vi "Advanced Cut - Remove Snippet Impulse Data.vi"(8 "error in (no error)":errorcluster, 10 "Snippet Domain in (samples)":dbl[](array[numeric]), 11 "Data IN":T1={"Impulse Positions"=[], "No. Imp"=0, "Parameter Time Series"=[], "Parameter Impuls Series"=[], "Experiment Parameters"={"Freq"=0.0, "Vel"=0, "Acc"=0, "Stimulus"=""}, "Autosort File"=refnum, "Data File"={"Data Channels"=[], "Sample Rate"=0, "Channel List"=[]}, "Experiment data path"=path "/Macintosh HD/Users/patrick/Studium/Diploma Thesis/Data Analysis", "Image data path"=path "/Macintosh HD/Users/patrick/Studium/Diploma Thesis/Data Analysis", "LVS data path"=path "/Macintosh HD/Users/patrick/Studium/Diploma Thesis/Data Analysis", "Raw copy path"=path "/Macintosh HD/Users/patrick/Studium/Diploma Thesis/Data Analysis", "filename"="No file selected", "desaccading parameters"={"Tolerance"=0, "Acc Range"=0.0, "Sample Rate"=0, "Impulse Plane 2"=enum."Other", "Impulse dir"=FALSE}, "Experiment Parameters 2"={"Subject"="", "Strain"="", "Rotation plane"="", "Experimenter"="", "Trial"=0.0, "Time"=0.0}, "Excel"={"Excel._Application"=refnum, "Use Excel"=FALSE, "Worksheet SINE"=refnum, "Row SINE"=0, "Worksheet TRANS"=refnum, "Row TRANS"=0}, "Session Config File"=refnum, "Autosort Parameter Set"=1, "EMA Version"="", "desacc "={"Threshold 1 [Acc]"=7000.0, "Threshold 2 [% of TH1]"=60, "tolerance"=3, "Search WD "=0.1, " always use TH2"=FALSE, "Range"=2.0, "Max time"=120.0, "Min time"=20.0, "Velocity Threshold"=150}, "Cycle Nr for Saccades"={"POS"=0, "NEG"=0}, "calibration name"="No file selected"} {"Parameter Time Series"."time offset" format="%.3f"; "Parameter Time Series"."Gain" format="%.1f"; "Parameter Time Series"."Offset" format="%.1f"; "Parameter Time Series"."List 1" items=["Motor-Pos", "Motor-Vel", "Lx Position-in-Head", "Ly Position-in-Head", "Lz Position-in-Head", "Lx Velocity-in-Head", "Ly Velocity-in-Head", "Lz Velocity-in-Head", "Ll Velocity-in-Head", "Lr Velocity-in-Head", "Lx Accel-in-Head", "Ly Accel-in-Head", "Lz Accel-in-Head", "Rx Position-in-Head", "Ry Position-in-Head", "Rz Position-in-Head", "Rx Velocity-in-Head", "Ry Velocity-in-Head", "Rz Velocity-in-Head", "Rl Velocity-in-Head", "Rr Velocity-in-Head", "Rx Accel-in-Head", "Ry Accel-in-Head", "Rz Accel-in-Head", "Global Trigger", "", "", ""]; "Parameter Impuls Series"."Gain" format="%.1f"; "Parameter Impuls Series"."Offset" format="%.1f"}) -> (0 "error out":errorcluster, 2 "Snippet Domain out (samples)":dbl[](array[numeric]), 3 "Data OUT":T1={"Impulse Positions"=[], "No. Imp"=0, "Parameter Time Series"=[], "Parameter Impuls Series"=[], "Experiment Parameters"={"Freq"=0.0, "Vel"=0, "Acc"=0, "Stimulus"=""}, "Autosort File"=refnum, "Data File"={"Data Channels"=[], "Sample Rate"=0, "Channel List"=[]}, "Experiment data path"=path "/Macintosh HD/Users/patrick/Studium/Diploma Thesis/Data Analysis", "Image data path"=path "/Macintosh HD/Users/patrick/Studium/Diploma Thesis/Data Analysis", "LVS data path"=path "/Macintosh HD/Users/patrick/Studium/Diploma Thesis/Data Analysis", "Raw copy path"=path "/Macintosh HD/Users/patrick/Studium/Diploma Thesis/Data Analysis", "filename"="No file selected", "desaccading parameters"={"Tolerance"=0, "Acc Range"=0.0, "Sample Rate"=0, "Impulse Plane 2"=enum."Other", "Impulse dir"=FALSE}, "Experiment Parameters 2"={"Subject"="", "Strain"="", "Rotation plane"="", "Experimenter"="", "Trial"=0.0, "Time"=0.0}, "Excel"={"Excel._Application"=refnum, "Use Excel"=FALSE, "Worksheet SINE"=refnum, "Row SINE"=0, "Worksheet TRANS"=refnum, "Row TRANS"=0}, "Session Config File"=refnum, "Autosort Parameter Set"=1, "EMA Version"="", "desacc "={"Threshold 1 [Acc]"=7000.0, "Threshold 2 [% of TH1]"=60, "tolerance"=3, "Search WD "=0.1, " always use TH2"=FALSE, "Range"=2.0, "Max time"=120.0, "Min time"=20.0, "Velocity Threshold"=150}, "Cycle Nr for Saccades"={"POS"=0, "NEG"=0}, "calibration name"="No file selected"} {"Parameter Time Series"."time offset" format="%.3f"; "Parameter Time Series"."Gain" format="%.1f"; "Parameter Time Series"."Offset" format="%.1f"; "Parameter Time Series"."List 1" items=["Motor-Pos", "Motor-Vel", "Lx Position-in-Head", "Ly Position-in-Head", "Lz Position-in-Head", "Lx Velocity-in-Head", "Ly Velocity-in-Head", "Lz Velocity-in-Head", "Ll Velocity-in-Head", "Lr Velocity-in-Head", "Lx Accel-in-Head", "Ly Accel-in-Head", "Lz Accel-in-Head", "Rx Position-in-Head", "Ry Position-in-Head", "Rz Position-in-Head", "Rx Velocity-in-Head", "Ry Velocity-in-Head", "Rz Velocity-in-Head", "Rl Velocity-in-Head", "Rr Velocity-in-Head", "Rx Accel-in-Head", "Ry Accel-in-Head", "Rz Accel-in-Head", "Global Trigger", "", "", ""]; "Parameter Impuls Series"."Gain" format="%.1f"; "Parameter Impuls Series"."Offset" format="%.1f"})   [LabVIEW 2016]
uses:
  core/type-defs/TD_Statemachine-Data.ctl
  core/type-defs/TD_Time Series.ctl
  core/type-defs/TD_Impulse Parameter.ctl
  core/core.lvlib
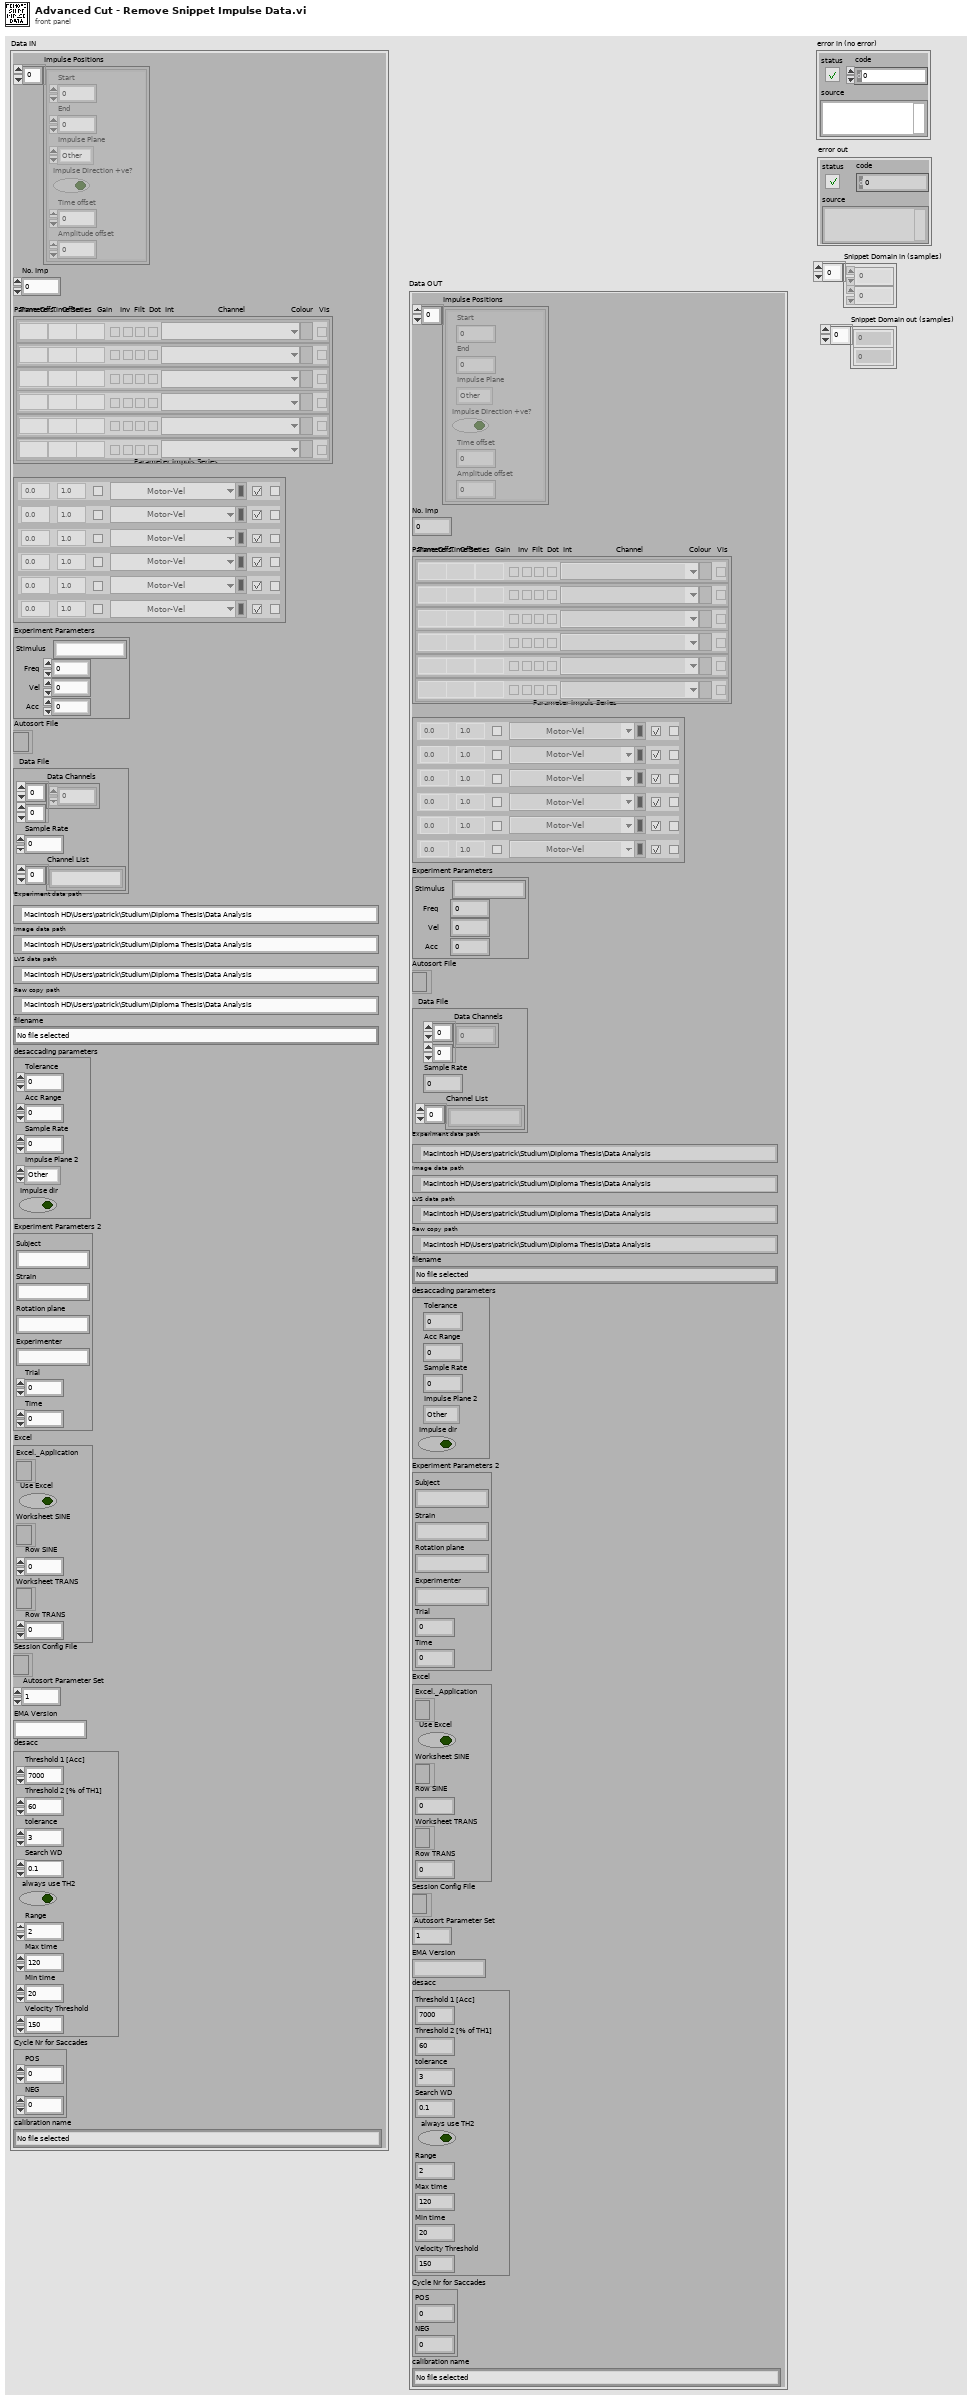
[diagram p1: front panel]
types:
  T1 = typedef "core.lvlib/TD_Statemachine-Data.ctl" = cluster{"Impulse Positions":cluster{"Start":i32, "End":i32, "Impulse Plane":enum16{"Other", "Yaw", "Pitch", "Roll", "LARP", "RALP"}, "Impulse Direction +ve?":bool, "Time offset":i32, "Amplitude offset":dbl}[], "No. Imp":i32, "Parameter Time Series":T2, "Parameter Impuls Series":T3, "Experiment Parameters":cluster{"Freq":dbl, "Vel":i32, "Acc":i32, "Stimulus":string}, "Autosort File":refnum<file>, "Data File":cluster{"Data Channels":dbl[][], "Sample Rate":i32, "Channel List":string[]}, "Experiment data path":path, "Image data path":path, "LVS data path":path, "Raw copy path":path, "filename":string, "desaccading parameters":cluster{"Tolerance":i32, "Acc Range":dbl, "Sample Rate":i32, "Impulse Plane 2":enum16{"Other", "Yaw", "Pitch", "Roll", "LARP", "RALP"}, "Impulse dir":bool}, "Experiment Parameters 2":cluster{"Subject":string, "Strain":string, "Rotation plane":string, "Experimenter":string, "Trial":dbl, "Time":dbl}, "Excel":cluster{"Excel._Application":refnum<k7>, "Use Excel":bool, "Worksheet SINE":refnum<k7>, "Row SINE":i32, "Worksheet TRANS":refnum<k7>, "Row TRANS":i32}, "Session Config File":refnum<file>, "Autosort Parameter Set":i32, "EMA Version":string, "desacc ":cluster{"Threshold 1 [Acc]":dbl, "Threshold 2 [% of TH1]":i32, "tolerance":i32, "Search WD ":dbl, " always use TH2":bool, "Range":dbl, "Max time":dbl, "Min time":dbl, "Velocity Threshold":i32}, "Cycle Nr for Saccades":cluster{"POS":i32, "NEG":i32}, "calibration name":string}
  T2 = typedef "core.lvlib/TD_Time Series.ctl" = cluster{"time offset":dbl, "Offset":dbl, "Gain":dbl, "inverse":bool, "filter data":bool, "dots":bool, "interpolate":bool, "List 1":u16, "Color Box":u32, "Boolean":bool}[]
  T3 = typedef "core.lvlib/TD_Impulse Parameter.ctl" = cluster{"Color":u32, "Visible":bool, "Channel":u16, "Invert":bool, "Desaccade":bool, "Offset":dbl, "Gain":dbl}[]
  T4 = cluster{"Start":i32, "End":i32, "Impulse Plane":enum16{"Other", "Yaw", "Pitch", "Roll", "LARP", "RALP"}, "Impulse Direction +ve?":bool, "Time offset":i32, "Amplitude offset":dbl}[]
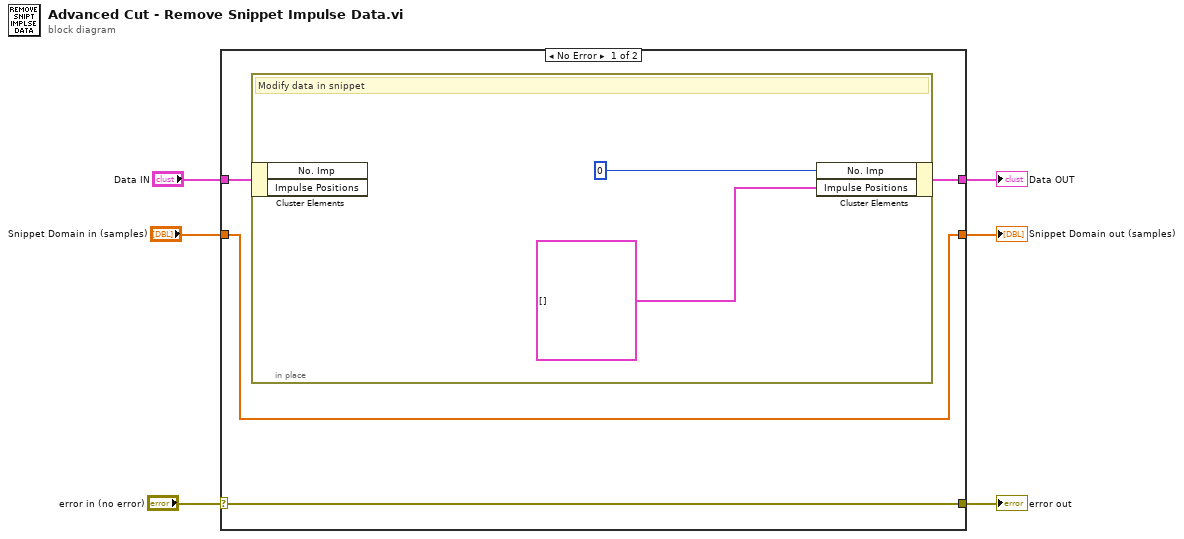
[diagram p0: block diagram]
diagram:
  n1 = case shown="No Error" "error in (no error)" {
    selector: "error in (no error)" -> [w8 w13]
    tunnel: "Data IN" -> [w10 w14]
    tunnel: "Snippet Domain in (samples)" -> [w7 w15]
    tunnel: [w9 w14] -> w2
    tunnel: [w8 w13] -> w3
    tunnel: [w7 w15] -> w1
    frame No Error {
      n2 = in-place {
        # "Modify data in snippet"
        n3 = in-place-cluster #1(w10) -> ()  [unwired: 2 out]
        n4 = in-place-cluster #1("No. Imp"=0, "Impulse Positions"=T4 []) -> (w9:T1)
      }
    }
    frame Error {
    }
  }
  "Data OUT" <- w2
  "error out" <- w3
  "Snippet Domain out (samples)" <- w1
